vi "SelectChassis.vi"(8 "error in":errorcluster, 10 "Chassis Alias List in":string[](array[string]), 11 "Chassis List in":string[](array[string])) -> (0 "error out":errorcluster)   [LabVIEW 2011]
doc: "This VI will ask user to select cDAQ Chassis."
panel:
  out "Selection":string
  out "Cancelled?":bool
  in  "Cancel":bool
  in  "Done":bool
  in  "Listbox":i32(listbox)=1
  # "Please select your CompactDAQ Chassis from the list..."
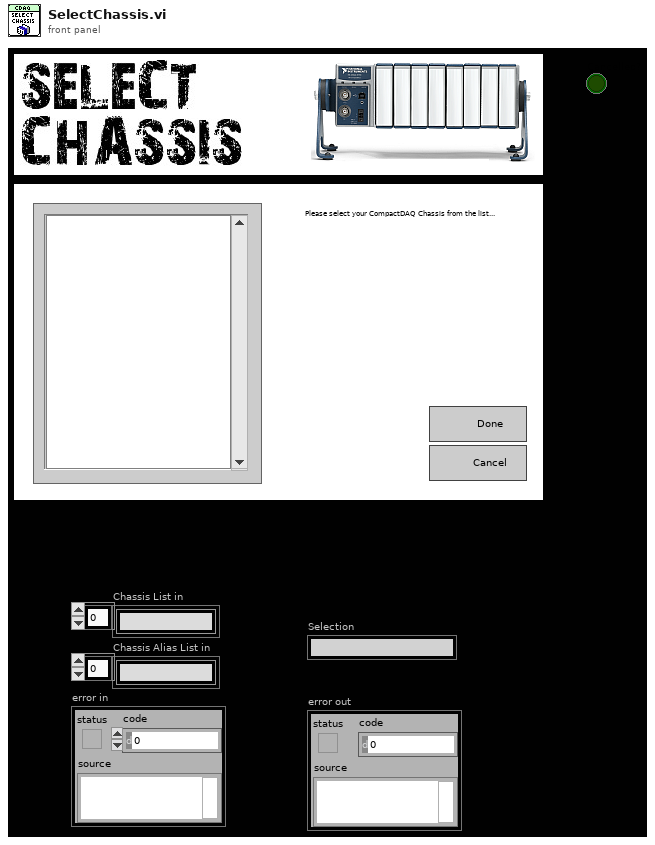
[diagram p1: front panel]
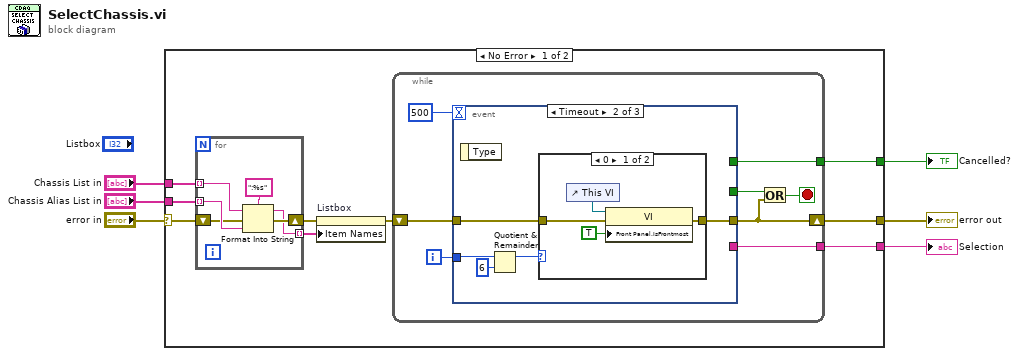
[diagram p0: block diagram]
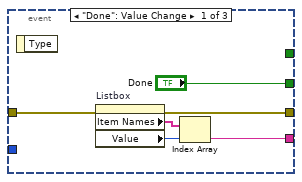
[diagram p2: hidden frame]
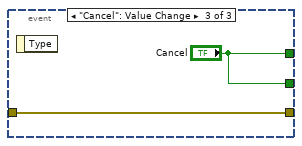
[diagram p4: hidden frame]
diagram:
  n1 = case shown="No Error" "error in" {
    selector: "error in" -> [w7 w48]
    tunnel: "Chassis List in" -> [w15 _]
    tunnel: "Chassis Alias List in" -> [w14 _]
    tunnel: [w10 w48] -> w4
    tunnel: [w9 _] -> w3
    tunnel: [w8 _] -> w2
    frame No Error {
      n2 = for {
        tunnel: w15 -> [w46] mode=indexing
        tunnel: w14 -> [w45] mode=indexing
        shift-right: [w44] -> w13
        shift-left: w7 -> [w43]
        tunnel: [w42] -> w12 mode=indexing
        n3 = Format Into String(format string=":%s", initial string=w46, error in=w43, w45) -> (resulting string=w42:string, error out=w44:errorcluster)
      }
      n4 = property on="Listbox" class="LstBox (strict)"(error in=w13, "Item Names"=w12) -> (error out=w11:errorcluster)  [unwired: 1 in, 1 out]
      n5 = while {
        shift-right: [w22] -> w10
        shift-left: w11 -> [w23]
        tunnel: [w19] -> w9
        tunnel: [w18] -> w8
        i -> [w16]
        stop <- w21 stop-if-true
        n6 = event shown="[1] Timeout" {
          selector: _ -> [_ _ _]
          dyn-events: _ -> [_ _ _]
          timeout: 500 -> [_ _ _]
          tunnel: w23 -> [w28 w34 w40]
          tunnel: [w24 w33 w40] -> w22
          tunnel: ["Done" _ "Cancel"] -> w20
          tunnel: [_ _ "Cancel"] -> w19
          tunnel: [w25 _ _] -> w18
          tunnel: w16 -> [_ w32 _]
          event "Done": Value Change {
            n7 = event-data() -> ()  [unwired: 1 in, 1 out]
            n8 = property on="Listbox" class="LstBox (strict)"(error in=w28) -> (error out=w24:errorcluster, "Item Names"=w27:string[], "Value"=w26:i32)  [unwired: 1 in, 1 out]
            n9 = Index Array(array=w27, index=w26) -> (element=w25:string)
          }
          event Timeout {
            n10 = event-data() -> ()  [unwired: 1 in, 1 out]
            n11 = Quotient & Remainder(x=w32, y=6) -> (x-y*floor(x/y)=w30:i32)  [unwired: 1 out]
            n12 = case shown="0" w30 {
              tunnel: w34 -> [w37 w39]
              tunnel: [w38 w39] -> w33
              frame 0 {
                n13 = control-ref of="This VI"() -> (w36:refnum<vi>)
                n14 = property class="VI"(reference=w36, error in=w37, "Front Panel.IsFrontmost"=TRUE ("Front Panel Window:Is Frontmost")) -> (error out=w38:errorcluster)  [unwired: 1 out]
              }
              frame Default {
              }
            }
          }
          event "Cancel": Value Change {
            n15 = event-data() -> ()  [unwired: 1 in, 1 out]
          }
        }
        n16 = Or(x=w20, y=w22) -> (x .or. y?=w21:bool)
      }
    }
    frame Error {
    }
  }
  "error out" <- w4
  "Cancelled?" <- w3
  "Selection" <- w2
